vi "Shooter Controller.vi"(8 "error in (no error)":errorcluster) -> ()   [LabVIEW 2016]
uses:
  <vilib>/Rock Robotics/WPI/MotorControl/WPI_MotorControlDeviceRef.ctl
  <vilib>/Rock Robotics/WPI/MotorControl/WPI_MotorControlType.ctl
  <vilib>/Rock Robotics/SystemInterfaces/DIO/FPGA_DIOPWMChannel.ctl
  <vilib>/Rock Robotics/WPI/PWM/WPI_PWMDeadband.ctl
  Shooterqueue.ctl
panel:
  out "RPM:":dbl
  in  "Stop":bool
  in  "Speed":dbl(slide) caption="Debug Set Speed (Continuous)" scale=0.0..8000.0
  in  "Feeder PIDF":cluster{"Kp":dbl, "Ki":dbl, "Kd":dbl, "Kf":dbl}={"Kp"=0.0008, "Ki"=1e-05, "Kd"=0.015, "Kf"=0.000216} {"Kf" format="%.6f"; "Kd" format="%.6f"; "Ki" format="%.6f"; "Kp" format="%.6f"}
  in  "Set":bool
  in  "IZone":dbl=2000.0 format="%.2f"
  in  "Shooter PIDF":cluster{"Kp":dbl, "Ki":dbl, "Kd":dbl, "Kf":dbl}={"Kp"=0.16, "Ki"=0.0015, "Kd"=10.0, "Kf"=0.065} {"Kf" format="%.6f"; "Kd" format="%.6f"; "Ki" format="%.6f"; "Kp" format="%.6f"}
  in  "Debug":enum16{"Feeder", "Rear", "Front", "None"}(ring)=enum."None"
  out "Waveform Chart":T1(graph)
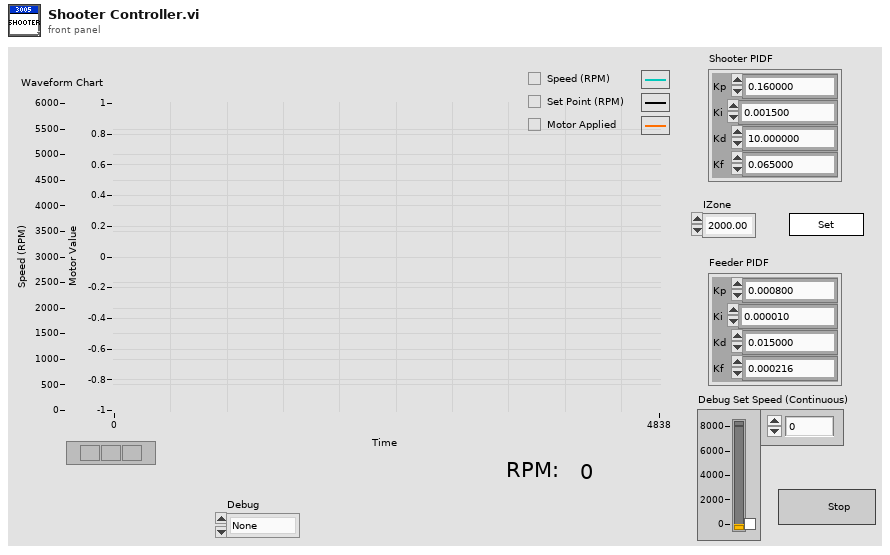
[diagram p1: front panel]
types:
  T1 = cluster{"Sensor Velocity":dbl, "Motor Output":dbl, "Applied Throttle":dbl}
  T2 = typedef "Shooterqueue.ctl" = cluster{"msg":string, "value":dbl}
  T3 = typedef "WPI_MotorControlDeviceRef.ctl" = cluster{"DeviceStatus":errorcluster, "Type":T4, "PWM":cluster{"PWM Channel":T5, "DeadBand":T6}, "CAN":cluster{"Device Number":u8, "SetOutput VI Ref":variant, "GetOutput VI Ref":variant, "Enable VI Ref":variant, "Disable VI Ref":variant, "Data":variant}, "Invert":bool}
  T4 = typedef "WPI_MotorControlType.ctl" = enum16{"PWM", "CAN"}
  T5 = typedef "FPGA_DIOPWMChannel.ctl" = enum8{"PWM 0", "PWM 1", "PWM 2", "PWM 3", "PWM 4", "PWM 5", "PWM 6", "PWM 7", "PWM 8", "PWM 9", "PWM MXP 0", "PWM MXP 1", "PWM MXP 2", "PWM MXP 3", "PWM MXP 4", "PWM MXP 5", "PWM MXP 6", "PWM MXP 7", "PWM MXP 8", "PWM MXP 9", "Invalid"}
  T6 = typedef "WPI_PWMDeadband.ctl" = cluster{"Name":string, "maxPositivePwm":i32, "minPositivePwm":i32, "centerPwm":i32, "maxNegativePwm":i32, "minNegativePwm":i32, "angularRange":u16}
  T7 = cluster{"Shooter Front":T3, "Shooter Rear":T3, "Feeder":T3, "Agitator":T3, "Front":dbl, "Rear":dbl, "Feeder":dbl, "queue":refnum<queue>}
  T8 = typedef "WPI_CANTalonSRX_GlobalStatus.ctl" = cluster{"Applied Throttle":dbl, "Module Enabled":bool, "CAN Error":errorcluster, "Closed Loop Error":dbl, "Forward Limit Switch Closed":bool, "Reverse Limit Switch Closed":bool, "Sensor Position":dbl, "Sensor Velocity":dbl, "Current":dbl, "Sticky Fault - Over Temp":bool, "Sticky Fault - Under Voltage":bool, "Sticky Fault - Forward Limit":bool, "Sticky Fault - Reverse Limit":bool, "Sticky Fault - Forward Soft Limit":bool, "Sticky Fault - Reverse Soft Limit":bool, "Brake is Enabled":bool, "Encoder Position":dbl, "Encoder Velocity":dbl, "Encoder Index Count":dbl, "Encoder A Pin State":bool, "Encoder B Pin State":bool, "Encoder Index Pin State":bool, "Analog In":dbl, "Analog In Velocity":dbl, "Temperature (C)":dbl, "Battery Voltage":dbl, "Control 5 Is Supported":bool, "Current Profile Slot Select":dbl, "Pos Div 8":bool, "Vel Div 4":bool, "Pulse Width Position":i32, "Pulse Width Velocity":i32, "Pulse Width Rise To Rise (us)":i32, "Pulse Width Rise To Fall (us)":i32, "Mot Prof Active Is Under Run":bool, "Mot Prof Active Has Under Run":bool, "Mot Prof Active Is Last":bool, "Mot Prof Active Velocity Only":bool, "Mot Prof Active Is Valid":bool, "Mot Prof Buffer Is Full":bool, "Mot Prof Active Profile Slot Select":i32, "Mot Prof NextID":i32, "Mot Prof Count":i32, "Mot Prof Active Velocity":dbl, "Mot Prof Active Position":dbl, "Mot Prof Output Enable":i32, "UsageFrame":u32, "Motion Magic Active Trajectory":cluster{"Velocity":dbl, "Position":dbl}}
  T9 = cluster{"Sensor Velocity":dbl, "Output":dbl, "Applied Throttle":dbl}
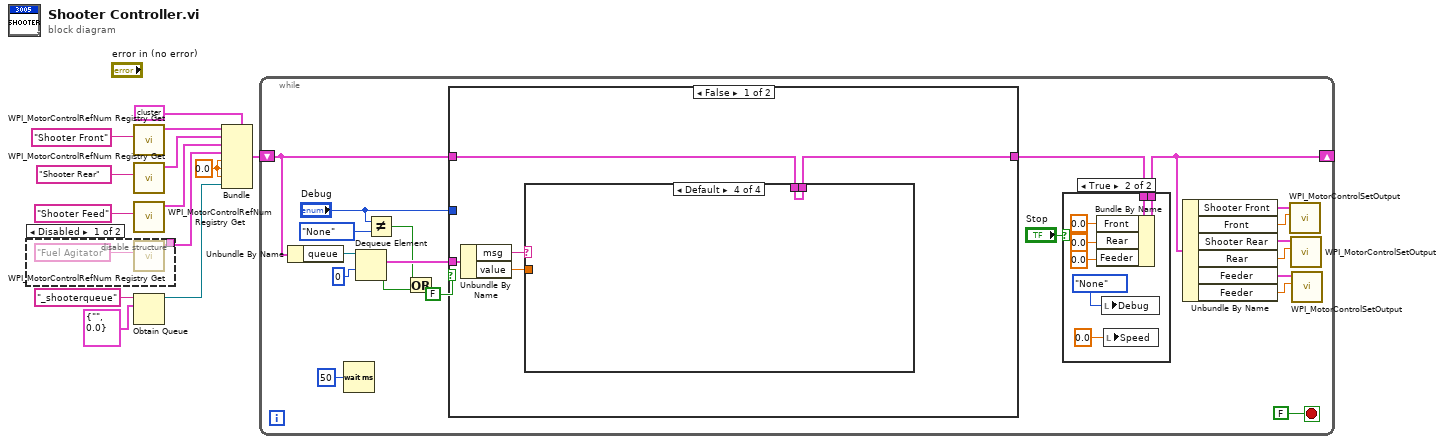
[diagram p0: block diagram]
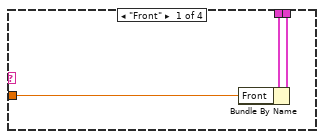
[diagram p3: hidden frame]
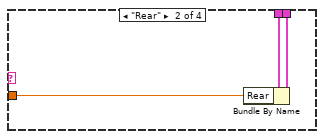
[diagram p4: hidden frame]
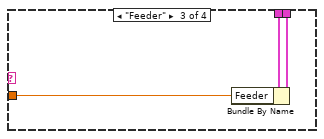
[diagram p5: hidden frame]
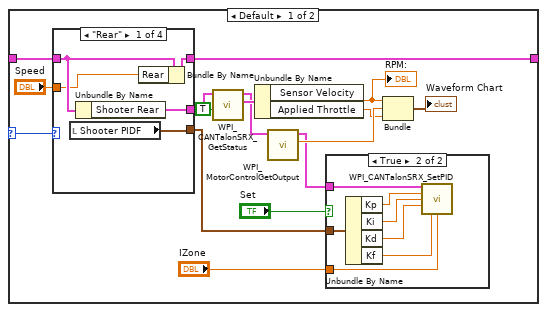
[diagram p7: hidden frame]
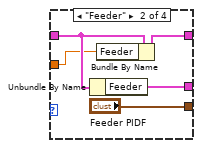
[diagram p8: hidden frame]
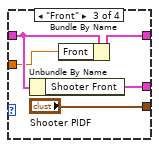
[diagram p9: hidden frame]
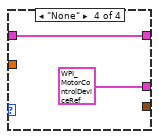
[diagram p10: hidden frame]
diagram:
  w3 = 0.0 ("Rear")
  n1 = disable-structure shown="Disabled" {
    disable-tunnel: [w15 _] -> w13
    frame Disabled {
      n2 = call <vilib>:"WPI_MotorControlRefNum Registry Get.vi"("refnum name"="Fuel Agitator") -> ("MotorControlDevRef"=w15:T3)  [unwired: 9 in, 1 out]
    }
    frame Enabled {
    }
  }
  n3 = call <vilib>:"WPI_MotorControlRefNum Registry Get.vi"("refnum name"="Shooter Front") -> ("MotorControlDevRef"=w10:T3)  [unwired: 9 in, 1 out]
  n4 = call <vilib>:"WPI_MotorControlRefNum Registry Get.vi"("refnum name"="Shooter Rear") -> ("MotorControlDevRef"=w11:T3)  [unwired: 9 in, 1 out]
  n5 = call <vilib>:"WPI_MotorControlRefNum Registry Get.vi"("refnum name"="Shooter Feed") -> ("MotorControlDevRef"=w12:T3)  [unwired: 9 in, 1 out]
  n6 = Obtain Queue(name (unnamed)="_shooterqueue", element data type=T2 {"msg"="", "value"=0.0}) -> (queue out=w1:refnum<queue>)  [unwired: 3 in, 2 out]
  n7 = Bundle(cluster=T7 {"Shooter Front"={"DeviceStatus"={"status"=FALSE, "code"=0, "source"=""}, "Type"=enum."PWM", "PWM"={"PWM Channel"=enum."PWM 0", "DeadBand"={"Name"="", "maxPositivePwm"=0, "minPositivePwm"=0, "centerPwm"=0, "maxNegativePwm"=0, "minNegativePwm"=0, "angularRange"=0}}, "CAN"={"Device Number"=0, "SetOutput VI Ref"=variant, "GetOutput VI Ref"=variant, "Enable VI Ref"=variant, "Disable VI Ref"=variant, "Data"=variant}, "Invert"=FALSE}, "Shooter Rear"={"DeviceStatus"={"status"=FALSE, "code"=0, "source"=""}, "Type"=enum."PWM", "PWM"={"PWM Channel"=enum."PWM 0", "DeadBand"={"Name"="", "maxPositivePwm"=0, "minPositivePwm"=0, "centerPwm"=0, "maxNegativePwm"=0, "minNegativePwm"=0, "angularRange"=0}}, "CAN"={"Device Number"=0, "SetOutput VI Ref"=variant, "GetOutput VI Ref"=variant, "Enable VI Ref"=variant, "Disable VI Ref"=variant, "Data"=variant}, "Invert"=FALSE}, "Feeder"={"DeviceStatus"={"status"=FALSE, "code"=0, "source"=""}, "Type"=enum."PWM", "PWM"={"PWM Channel"=enum."PWM 0", "DeadBand"={"Name"="", "maxPositivePwm"=0, "minPositivePwm"=0, "centerPwm"=0, "maxNegativePwm"=0, "minNegativePwm"=0, "angularRange"=0}}, "CAN"={"Device Number"=0, "SetOutput VI Ref"=variant, "GetOutput VI Ref"=variant, "Enable VI Ref"=variant, "Disable VI Ref"=variant, "Data"=variant}, "Invert"=FALSE}, "Agitator"={"DeviceStatus"={"status"=FALSE, "code"=0, "source"=""}, "Type"=enum."PWM", "PWM"={"PWM Channel"=enum."PWM 0", "DeadBand"={"Name"="", "maxPositivePwm"=0, "minPositivePwm"=0, "centerPwm"=0, "maxNegativePwm"=0, "minNegativePwm"=0, "angularRange"=0}}, "CAN"={"Device Number"=0, "SetOutput VI Ref"=variant, "GetOutput VI Ref"=variant, "Enable VI Ref"=variant, "Disable VI Ref"=variant, "Data"=variant}, "Invert"=FALSE}, "Front"=0.0, "Rear"=0.0, "Feeder"=0.0, "queue"=refnum}, "Shooter Front"=w10, "Shooter Rear"=w11, "Feeder"=w12, "Agitator"=w13, "Front"=w3, "Rear"=w3, "Feeder"=w3, "queue"=w1) -> (w9:T7)
  n8 = while {
    shift-right: [w21] -> _
    shift-left: w9 -> [w26]
    stop <- FALSE ("stop") stop-if-true
    n9 = Unbundle By Name(w26) -> ("queue"=w25:refnum<queue>)
    n10 = Wait (ms)(milliseconds to wait=u32 50) -> ()  [unwired: 1 out]
    n11 = Dequeue Element(queue=w25, timeout in ms (-1)=0) -> (element=w23:T2, timed out?=w24:bool)  [unwired: 1 in, 2 out]
    n12 = Not Equal?(x="Debug", y=enum16{"Feeder", "Rear", "Front", "None"}."None") -> (x != y?=w17:bool)
    n13 = Or(x=w17, y=w24) -> ()  [unwired: 1 out]
    n14 = case shown="False" FALSE {
      tunnel: w26 -> [w46 w61]
      tunnel: [w45 w60] -> w34
      tunnel: w23 -> [w48 _]
      tunnel: "Debug" -> [_ w59]
      frame False {
        n15 = Unbundle By Name(w48) -> ("msg"=w47:string, "value"=w44:dbl)
        n16 = case shown="Default" w47 {
          tunnel: w46 -> [w51 w54 w57 w58]
          tunnel: [w50 w53 w56 w58] -> w45
          tunnel: w44 -> [w49 w52 w55 _]
          frame "Front" {
            n17 = Bundle By Name(cluster=w51, "Front"=w49) -> (w50:T7)
          }
          frame "Rear" {
            n18 = Bundle By Name(cluster=w54, "Rear"=w52) -> (w53:T7)
          }
          frame "Feeder" {
            n19 = Bundle By Name(cluster=w57, "Feeder"=w55) -> (w56:T7)
          }
          frame Default {
          }
        }
      }
      frame True {
        n20 = case shown="\"None\"" w59 {
          selector: w59 -> [w77 _]
          tunnel: w61 -> [w76 w102]
          tunnel: [w75 w102] -> w60
          frame Default {
            n21 = case shown="\"Rear\"" w77 {
              tunnel: w76 -> [w82 w87 w92 w94]
              tunnel: [w79 w84 w89 w94] -> w75
              tunnel: [w81 w86 w91 T3 {"DeviceStatus"={"status"=FALSE, "code"=0, "source"=""}, "Type"=enum."PWM", "PWM"={"PWM Channel"=enum."Invalid", "DeadBand"={"Name"="", "maxPositivePwm"=0, "minPositivePwm"=0, "centerPwm"=0, "maxNegativePwm"=0, "minNegativePwm"=0, "angularRange"=0}}, "CAN"={"Device Number"=0, "SetOutput VI Ref"=variant, "GetOutput VI Ref"=variant, "Enable VI Ref"=variant, "Disable VI Ref"=variant, "Data"=variant}, "Invert"=FALSE} ("Shooter Front")] -> w74
              tunnel: [w80 "Feeder PIDF" "Shooter PIDF" _] -> w66
              tunnel: "Speed" -> [w78 w83 w88 _]
              frame "Rear" {
                n22 = local read "Shooter PIDF"() -> (w80:cluster{"Kp":dbl, "Ki":dbl, "Kd":dbl, "Kf":dbl})
                n23 = Unbundle By Name(w82) -> ("Shooter Rear"=w81:T3)
                n24 = Bundle By Name(cluster=w82, "Rear"=w78) -> (w79:T7)
              }
              frame "Feeder" {
                n25 = Unbundle By Name(w87) -> ("Feeder"=w86:T3)
                n26 = Bundle By Name(cluster=w87, "Feeder"=w83) -> (w84:T7)
              }
              frame "Front" {
                n27 = Unbundle By Name(w92) -> ("Shooter Front"=w91:T3)
                n28 = Bundle By Name(cluster=w92, "Front"=w88) -> (w89:T7)
              }
              frame "None" {
              }
            }
            n29 = call <vilib>:"WPI_CANTalonSRX_GetStatus.vi"("Clear Sticky Faults"=TRUE, "CAN Talon SRX Ref"=w74) -> ("Talon SRX Status"=w73:T8, "CAN Talon SRX Ref"=w72:T3)  [unwired: 7 in, 1 out]
            n30 = Unbundle By Name(w73) -> ("Sensor Velocity"=w63:dbl, "Applied Throttle"=w65:dbl)
            "RPM:" <- w63
            n31 = call <vilib>:"WPI_MotorControlGetOutput.vi"("MotorControlDevRef"=w72) -> ("Output"=w71:dbl, "MotorControlDevRef"=w68:T3)  [unwired: 8 in, 1 out]
            n32 = case shown="True" "Set" {
              tunnel: "IZone" -> [_ w97]
              tunnel: w66 -> [_ w96]
              tunnel: w68 -> [_ w95]
              frame False {
              }
              frame True {
                n33 = Unbundle By Name(w96) -> ("Kp"=w101:dbl, "Ki"=w100:dbl, "Kd"=w99:dbl, "Kf"=w98:dbl)
                n34 = call <vilib>:"WPI_CANTalonSRX_SetPID.vi"("CAN Talon SRX Ref"=w95, "P"=w101, "I"=w100, "D"=w99, "F"=w98, "I Zone"=w97) -> ()  [unwired: 8 in, 2 out]
              }
            }
            n35 = Bundle("Sensor Velocity"=w63, "Output"=w71, "Applied Throttle"=w65) -> (→"Waveform Chart":T9)  [unwired: 1 in]
          }
          frame "None" {
          }
        }
      }
    }
    n36 = case shown="True" "Stop" {
      tunnel: w34 -> [w36 w43]
      tunnel: [w36 w42] -> w21
      frame False {
      }
      frame True {
        n37 = Bundle By Name(cluster=w43, "Front"=0.0, "Rear"=0.0, "Feeder"=0.0) -> (w42:T7)
        n38 = local write "Debug"(enum16{"Feeder", "Rear", "Front", "None"}."None" ("Debug")) -> ()
        n39 = local write "Speed"(0.0 ("Speed")) -> ()
      }
    }
    n40 = Unbundle By Name(w21) -> ("Shooter Front"=w33:T3, "Front"=w32:dbl, "Shooter Rear"=w31:T3, "Rear"=w30:dbl, "Feeder"=w29:T3, "Feeder"=w28:dbl)
    n41 = call <vilib>:"WPI_MotorControlSetOutput.vi"("Output"=w32, "MotorControlDevRef"=w33) -> ()  [unwired: 7 in, 3 out]
    n42 = call <vilib>:"WPI_MotorControlSetOutput.vi"("Output"=w30, "MotorControlDevRef"=w31) -> ()  [unwired: 7 in, 3 out]
    n43 = call <vilib>:"WPI_MotorControlSetOutput.vi"("Output"=w28, "MotorControlDevRef"=w29) -> ()  [unwired: 7 in, 3 out]
  }
